vi "QCA - Initialize DUT For AR9880.vi"(8 "error in (no error)":errorcluster, 11 "index":i32) -> (0 "error out":errorcluster, 1 "CmdCount":i32, 2 "Cmd":string, 3 "Command List":string[](array[string]))   [LabVIEW 2012]
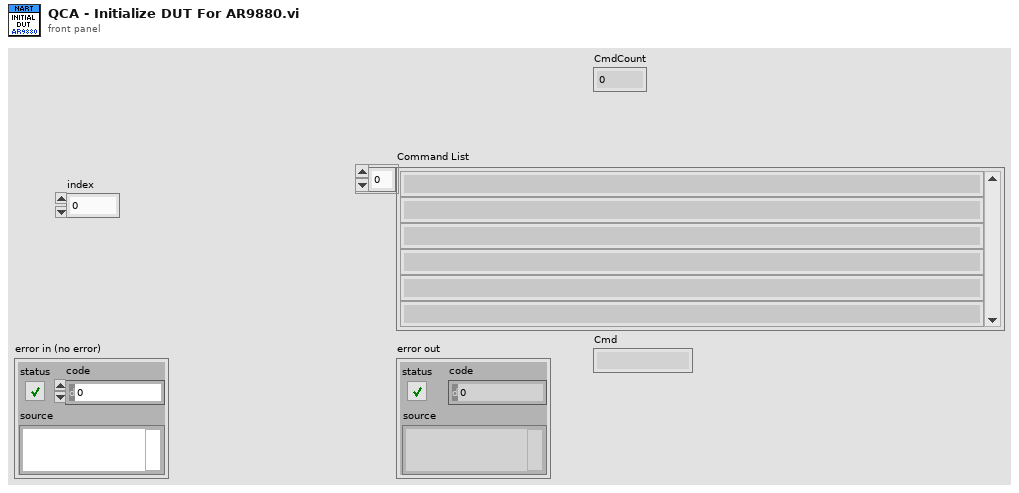
[diagram p1: front panel]
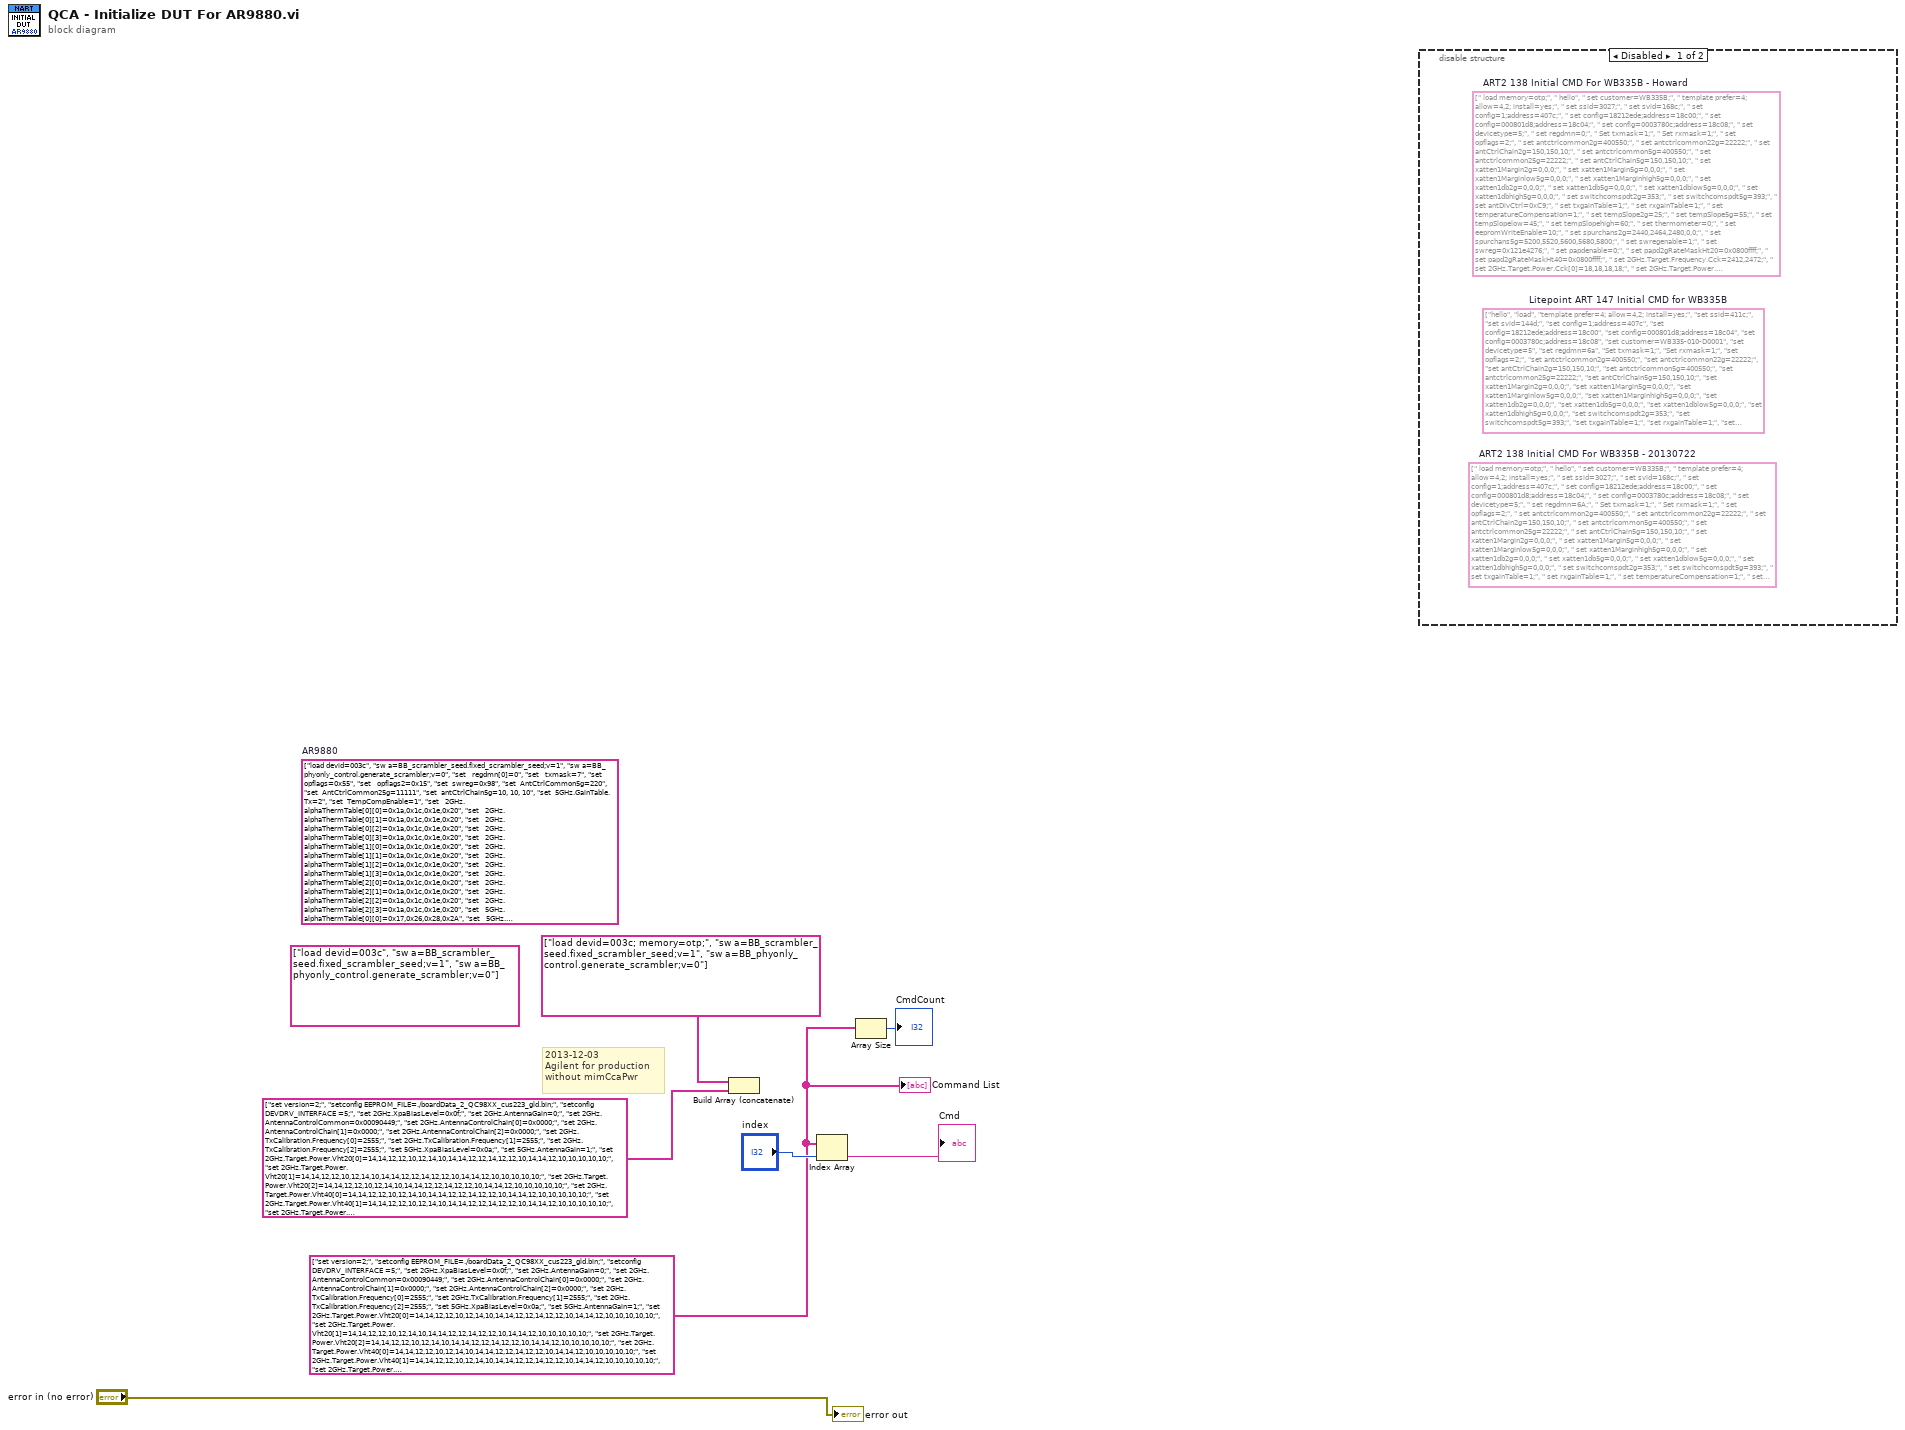
[diagram p0: block diagram]
diagram:
  w1 = string[] ["set version=2;", "setconfig EEPROM_FILE=./boardData_2_QC98XX_cus223_gld.bin;", "setconfig DEVDRV_INTERFACE =5;", "set 2GHz.XpaBiasLevel=0x0f;", "set 2GHz.AntennaGain=0;", "set 2GHz.AntennaControlCommon=0x00090449;", "set 2GHz.AntennaControlChain[0]=0x0000;", "set 2GHz.AntennaControlChain[1]=0x0000;", "set 2GHz.AntennaControlChain[2]=0x0000;", "set 2GHz.TxCalibration.Frequency[0]=2555;", "set 2GHz.TxCalibration.Frequency[1]=2555;", "set 2GHz.TxCalibration.Frequency[2]=2555;", "set 5GHz.XpaBiasLevel=0x0a;", "set 5GHz.AntennaGain=1;", "set 2GHz.Target.Power.Vht20[0]=14,14,12,12,10,12,14,10,14,14,12,12,14,12,12,10,14,14,12,10,10,10,10,10;", "set 2GHz.Target.Power.Vht20[1]=14,14,12,12,10,12,14,10,14,14,12,12,14,12,12,10,14,14,12,10,10,10,10,10;", "set 2GHz.Target.Power.Vht20[2]=14,14,12,12,10,12,14,10,14,14,12,12,14,12,12,10,14,14,12,10,10,10,10,10;", "set 2GHz.Target.Power.Vht40[0]=14,14,12,12,10,12,14,10,14,14,12,12,14,12,12,10,14,14,12,10,10,10,10,10;", "set 2GHz.Target.Power.Vht40[1]=14,14,12,12,10,12,14,10,14,14,12,12,14,12,12,10,14,14,12,10,10,10,10,10;", "set 2GHz.Target.Power.Vht40[2]=14,14,12,12,10,12,14,10,14,14,12,12,14,12,12,10,14,14,12,10,10,10,10,10;", "set regdmn[0]=0;", "set txmask=7;", "set rxmask=7;", "set opflags=0x55;", "set opflags2=0x15;", "set swreg=0x98;", "set AntCtrlCommon5g=220;", "set AntCtrlCommon25g=11111;", "set antCtrlChain5g=10,10,10;", "set 5GHz.GainTable.Tx=2;", "set 5GHz.GainTable.Rx=0;", "set TempCompEnable=1;", "set 2GHz.alphaThermTable[0][0]=0x1a,0x1c,0x1e,0x20;", "set 2GHz.alphaThermTable[0][1]=0x1a,0x1c,0x1e,0x20;", "set 2GHz.alphaThermTable[0][2]=0x1a,0x1c,0x1e,0x20;", "set 2GHz.alphaThermTable[0][3]=0x1a,0x1c,0x1e,0x20;", "set 2GHz.alphaThermTable[1][0]=0x1a,0x1c,0x1e,0x20;", "set 2GHz.alphaThermTable[1][1]=0x1a,0x1c,0x1e,0x20;", "set 2GHz.alphaThermTable[1][2]=0x1a,0x1c,0x1e,0x20;", "set 2GHz.alphaThermTable[1][3]=0x1a,0x1c,0x1e,0x20;", "set 2GHz.alphaThermTable[2][0]=0x1a,0x1c,0x1e,0x20;", "set 2GHz.alphaThermTable[2][1]=0x1a,0x1c,0x1e,0x20;", "set 2GHz.alphaThermTable[2][2]=0x1a,0x1c,0x1e,0x20;", "set 2GHz.alphaThermTable[2][3]=0x1a,0x1c,0x1e,0x20;", "set 5GHz.alphaThermTable[0][0]=0x24,0x24,0x26,0x2C;", "set 5GHz.alphaThermTable[0][1]=0x24,0x24,0x26,0x2C;", "set 5GHz.alphaThermTable[0][2]=0x24,0x24,0x26,0x2C;", "set 5GHz.alphaThermTable[0][3]=0x24,0x24,0x26,0x2C;", "set 5GHz.alphaThermTable[0][4]=0x27,0x26,0x3D,0x3A;", "set 5GHz.alphaThermTable[0][5]=0x27,0x26,0x3D,0x3A;", "set 5GHz.alphaThermTable[0][6]=0x27,0x26,0x3D,0x3A;", "set 5GHz.alphaThermTable[0][7]=0x27,0x26,0x3D,0x3A;", "set 5GHz.alphaThermTable[1][0]=0x24,0x24,0x30,0x34;", "set 5GHz.alphaThermTable[1][1]=0x24,0x24,0x30,0x34;", "set 5GHz.alphaThermTable[1][2]=0x24,0x24,0x30,0x34;", "set 5GHz.alphaThermTable[1][3]=0x24,0x24,0x30,0x34;", "set 5GHz.alphaThermTable[1][4]=0x24,0x24,0x42,0x3E;", "set 5GHz.alphaThermTable[1][5]=0x24,0x24,0x42,0x3E;", "set 5GHz.alphaThermTable[1][6]=0x24,0x24,0x42,0x3E;", "set 5GHz.alphaThermTable[1][7]=0x24,0x24,0x42,0x3E;", "set 5GHz.alphaThermTable[2][0]=0x2B,0x2D,0x21,0x2E;", "set 5GHz.alphaThermTable[2][1]=0x2B,0x2D,0x21,0x2E;", "set 5GHz.alphaThermTable[2][2]=0x2B,0x2D,0x21,0x2E;", "set 5GHz.alphaThermTable[2][3]=0x2B,0x2D,0x21,0x2E;", "set 5GHz.alphaThermTable[2][4]=0x2C,0x2B,0x35,0x39;", "set 5GHz.alphaThermTable[2][5]=0x2C,0x2B,0x35,0x39;", "set 5GHz.alphaThermTable[2][6]=0x2C,0x2B,0x35,0x39;", "set 5GHz.alphaThermTable[2][7]=0x2C,0x2B,0x35,0x39;", "set FeatureEnable.TuningCaps=1;", "set TuningCaps=0x4f,0x4f;", "set antctrlchain5g=0x10;", "set 5GHz.Xatten1Db.Low =0x10,0x15,0x15;", "set 5GHz.Xatten1Db.Mid =0x12,0x15,0x12;", "set 5GHz.Xatten1Db.High =0x12,0x15,0x12;", "set 5GHz.Xatten1Margin.Low =0xa,0xa,0xa;", "set 5GHz.Xatten1Margin.Mid =0xa,0xa,0xa;", "set 5GHz.Xatten1Margin.High =0xa,0xa,0xa;", "set 5GHz.ctl.Index[0]=0x10;", "set 5GHz.ctl.Frequency[0]=5180,5260,5280,5500,5600,5700,5745,5825;", "set 5GHz.ctl.Power[0]=30.5  ,30.5  ,30.5  ,30.5  ,30.5  ,30.5  ,30.5  ,30;", "set 5GHz.ctl.BandEdge[0]=0   ,0   ,0   ,0   ,0   ,0   ,0   ,0;", "set 5GHz.ctl.Index[1]=0x16;", "set 5GHz.ctl.Frequency[1]=5180,5260,5280,5500,5520,5700,5745,5825;", "set 5GHz.ctl.Power[1]=30.5  ,30.5  ,30.5  ,30.5  ,30.5  ,30.5  ,30.5  ,30;", "set 5GHz.ctl.BandEdge[1]=0   ,0   ,0   ,0   ,0   ,0   ,0   ,0;", "set 5GHz.ctl.Index[2]=0x18;", "set 5GHz.ctl.Frequency[2]=5190,5230,5270,5310,5510,5550,5670,5755;", "set 5GHz.ctl.Power[2]=30  ,30.5  ,30  ,30.5  ,30.5  ,30.5  ,30.5  ,30.5;", "set 5GHz.ctl.BandEdge[2]=0   ,0   ,0   ,0   ,0   ,0   ,0   ,0;", "set 5GHz.ctl.Index[3]=0x19;", "set 5GHz.ctl.Frequency[3]=5180,5260,5280,5500,5520,5700,0,0;", "set 5GHz.ctl.Power[3]=30.5  ,30.5  ,30.5  ,30.5  ,30.5  ,30.5  ,0,0;", "set 5GHz.ctl.BandEdge[3]=0   ,0   ,0   ,0   ,0   ,0   ,0,0;", "set 5GHz.ctl.Index[6]=0x40;", "set 5GHz.ctl.Frequency[6]=5180,5200,5260,5320,5500,5700,6075,6075;", "set 5GHz.ctl.Power[6]=30  ,30.5  ,30.5  ,30  ,30.5  ,30  ,30  ,30;", "set 5GHz.ctl.BandEdge[6]=0   ,0   ,0   ,0   ,0   ,0   ,0   ,0;", "set 5GHz.ctl.Index[7]=0x46;", "set 5GHz.ctl.Frequency[7]=5180,5260,5500,5700,6075,6075,6075,6075;", "set 5GHz.ctl.Power[7]=30.5  ,30.5  ,30.5  ,30  ,30  ,30  ,30  ,30;", "set 5GHz.ctl.BandEdge[7]=0   ,0   ,0   ,0   ,0   ,0   ,0   ,0;", "set 5GHz.ctl.Index[8]=0x48;", "set 5GHz.ctl.Frequency[8]=5190,5270,5310,5510,5590,5670,6075,6075;", "set 5GHz.ctl.Power[8]=30.5  ,30.5  ,30.5  ,30.5  ,30.5  ,30  ,30  ,30;", "set 5GHz.ctl.BandEdge[8]=0   ,0   ,0   ,0   ,0   ,0   ,0   ,0;", "set 5GHz.ctl.Index[9]=0x49;", "set 5GHz.ctl.Frequency[9]=5180,5260,5500,5700,0,0,0,0;", "set 5GHz.ctl.Power[9]=30.5  ,30.5  ,30.5  ,30  ,0,0,0,0;", "set 5GHz.ctl.BandEdge[9]=0   ,0   ,0   ,0   ,0,0,0,0;", "set 5GHz.ctl.Index[12]=0x30;", "set 5GHz.ctl.Frequency[12]=5180,5200,5220,5260,5500,5600,5700,5745;", "set 5GHz.ctl.Power[12]=30.5  ,30.5  ,30.5  ,30.5  ,30.5  ,30.5  ,30.5  ,30.5;", "set 5GHz.ctl.BandEdge[12]=0   ,0   ,0   ,0   ,0   ,0   ,0   ,0;", "set 5GHz.ctl.Index[13]=0x36;", "set 5GHz.ctl.Frequency[13]=5180,5260,5320,5500,5560,5700,5745,5825;", "set 5GHz.ctl.Power[13]=30.5  ,30.5  ,30  ,30.5  ,30.5  ,30.5  ,30.5  ,30;", "set 5GHz.ctl.BandEdge[13]=0   ,0   ,0   ,0   ,0   ,0   ,0   ,0;", "set 5GHz.ctl.Index[14]=0x38;", "set 5GHz.ctl.Frequency[14]=5190,5230,5270,5510,5550,5670,5755,5795;", "set 5GHz.ctl.Power[14]=30.5  ,30  ,30.5  ,30.5  ,30.5  ,30.5  ,30  ,30.5;", "set 5GHz.ctl.BandEdge[14]=0   ,0   ,0   ,0   ,0   ,0   ,0   ,0;", "set 5GHz.ctl.Index[15]=0x39;", "set 5GHz.ctl.Frequency[15]=5180,5260,5320,5500,5560,5700,0,0;", "set 5GHz.ctl.Power[15]=30.5  ,30.5  ,30  ,30.5  ,30.5  ,30.5  ,0,0;", "set 5GHz.ctl.BandEdge[15]=0   ,0   ,0   ,0   ,0   ,0   ,0,0;", "set 5GHz.Target.Power.Legacy[0]=13.5,13.5,13.5,13.5;", "set 5GHz.Target.Power.Legacy[1]=13.5,13.5,13.5,13.5;", "set 5GHz.Target.Power.Legacy[2]=13.5,13.5,13.5,13.5;", "set 5GHz.Target.Power.Legacy[3]=19,18,17,17;", "set 5GHz.Target.Power.Legacy[4]=19,18,17,17;", "set 5GHz.Target.Power.Legacy[5]=19,18,17,17;", "set 5GHz.Target.Frequency.Vht20=5180,5240,5320,5500,5600,5745;", "set 5GHz.Target.Power.Vht20[0]=13.5,13.5,13.5,13.5,13.5,13.5,13.5,13.5,13.5,13.5,13.5,13.5,13.5,13.5,13.5,13.5,13.5,13.5,13.5,13.5,13.5,13.5,13.5,13.5;", "set 5GHz.Target.Power.Vht20[1]=13.5,13.5,13.5,13.5,13.5,13.5,13.5,13.5,13.5,13.5,13.5,13.5,13.5,13.5,13.5,13.5,13.5,13.5,13.5,13.5,13.5,13.5,13.5,13.5;", "set 5GHz.Target.Power.Vht20[2]=13.5,13.5,13.5,13.5,13.5,13.5,13.5,13.5,13.5,13.5,13.5,13.5,13.5,13.5,13.5,13.5,13.5,13.5,13.5,13.5,13.5,13.5,13.5,13.5;", "set 5GHz.Target.Power.Vht20[3]=19,19,18,17,17,16,14,14,19,19,18,17,17,16,14,14,19,19,18,17,17,16,14,14;", "set 5GHz.Target.Power.Vht20[4]=19,19,18,17,17,16,14,14,19,19,18,17,17,16,14,14,19,19,18,17,17,16,14,14;", "set 5GHz.Target.Power.Vht20[5]=19,19,18,17,17,16,14,14,19,19,18,17,17,16,14,14,19,19,18,17,17,16,14,14;", "set 5GHz.Target.Frequency.Vht40=5180,5240,5320,5500,5600,5745;", "set 5GHz.Target.Power.Vht40[0]=13.5,13.5,13.5,13.5,13.5,13.5,13.5,13.5,13.5,13.5,13.5,13.5,13.5,13.5,13.5,13.5,13.5,13.5,13.5,13.5,13.5,13.5,13.5,13.5;", "set 5GHz.Target.Power.Vht40[1]=13.5,13.5,13.5,13.5,13.5,13.5,13.5,13.5,13.5,13.5,13.5,13.5,13.5,13.5,13.5,13.5,13.5,13.5,13.5,13.5,13.5,13.5,13.5,13.5;", "set 5GHz.Target.Power.Vht40[2]=13.5,13.5,13.5,13.5,13.5,13.5,13.5,13.5,13.5,13.5,13.5,13.5,13.5,13.5,13.5,13.5,13.5,13.5,13.5,13.5,13.5,13.5,13.5,13.5;", "set 5GHz.Target.Power.Vht40[3]=19,19,18,17,17,16,14,14,19,19,18,17,17,16,14,14,19,19,18,17,17,16,14,14;", "set 5GHz.Target.Power.Vht40[4]=19,19,18,17,17,16,14,14,19,19,18,17,17,16,14,14,19,19,18,17,17,16,14,14;", "set 5GHz.Target.Power.Vht40[5]=19,19,18,17,17,16,14,14,19,19,18,17,17,16,14,14,19,19,18,17,17,16,14,14;", "set 5GHz.Target.Frequency.Vht80=5180,5240,5320,5500,5600,5745;", "set 5GHz.Target.Power.Vht80[0]=13.5,13.5,13.5,13.5,13.5,13.5,13.5,13.5,13.5,13.5,13.5,13.5,13.5,13.5,13.5,13.5,13.5,13.5,13.5,13.5,13.5,13.5,13.5,13.5;", "set 5GHz.Target.Power.Vht80[1]=13.5,13.5,13.5,13.5,13.5,13.5,13.5,13.5,13.5,13.5,13.5,13.5,13.5,13.5,13.5,13.5,13.5,13.5,13.5,13.5,13.5,13.5,13.5,13.5;", "set 5GHz.Target.Power.Vht80[2]=13.5,13.5,13.5,13.5,13.5,13.5,13.5,13.5,13.5,13.5,13.5,13.5,13.5,13.5,13.5,13.5,13.5,13.5,13.5,13.5,13.5,13.5,13.5,13.5;", "set 5GHz.Target.Power.Vht80[3]=19,19,18,17,17,16,14,14,19,19,18,17,17,16,14,14,19,19,18,17,17,16,14,14;", "set 5GHz.Target.Power.Vht80[4]=19,19,18,17,17,16,14,14,19,19,18,17,17,16,14,14,19,19,18,17,17,16,14,14;", "set 5GHz.Target.Power.Vht80[5]=19,19,18,17,17,16,14,14,19,19,18,17,17,16,14,14,19,19,18,17,17,16,14,14;", "setcal dll=cal-2p;", "setcal scheme=2;", "setcal PowerGoalMode=1;", "setcal 5gfreq=5180,5240,5320,5520,5640,5745,5785,5825;", "setcal 5gGainIndex1Ch0=9,9,9,9,9,9,10,10;", "setcal 5gGainIndex1Ch1=9,9,9,9,9,9,10,10;", "setcal 5gGainIndex1Ch2=9,9,9,9,9,9,10,10;", "setcal 5gDacGain1=0,0,0,0,0,0,0,0;", "setcal 5gPowerGoal1=14.0,14.0,14.0,14.0,14.0,14.0,14.0,14.0;", "setcal 5gGainIndex2Ch0=12,12,12,12,12,12,13,13;", "setcal 5gGainIndex2Ch1=12,12,12,12,12,12,13,13;", "setcal 5gGainIndex2Ch2=12,12,12,12,12,12,13,13;", "setcal 5gDacGain2=-6,-6,-6,-6,-6,-6,-6,-6;", "setcal 5gPowerGoal2=14.0,14.0,14.0,14.0,14.0,14.0,14.0,14.0;", "set customer=cus223-022-n0624;", "set 5GHz.Target.Frequency.Legacy[0]=5180;", "set 5GHz.Target.Frequency.Legacy[1]=5240;", "set 5GHz.Target.Frequency.Legacy[2]=5320;", "set 5GHz.Target.Frequency.Legacy[3]=5500;", "set 5GHz.Target.Frequency.Legacy[4]=5600;", "set 5GHz.Target.Frequency.Legacy[5]=5745;"] ("最终指令")
  (unwired) string[] ["load devid=003c", "sw a=BB_scrambler_seed.fixed_scrambler_seed;v=1", "sw a=BB_phyonly_control.generate_scrambler;v=0"]
  (unwired) string[] ["load devid=003c", "sw a=BB_scrambler_seed.fixed_scrambler_seed;v=1", "sw a=BB_phyonly_control.generate_scrambler;v=0", "set   regdmn[0]=0", "set   txmask=7", "set   opflags=0x55", "set   opflags2=0x15", "set  swreg=0x98", "set  AntCtrlCommon5g=220", "set  AntCtrlCommon25g=11111", "set  antCtrlChain5g=10, 10, 10", "set  5GHz.GainTable.Tx=2", "set  TempCompEnable=1", "set   2GHz.alphaThermTable[0][0]=0x1a,0x1c,0x1e,0x20", "set   2GHz.alphaThermTable[0][1]=0x1a,0x1c,0x1e,0x20", "set   2GHz.alphaThermTable[0][2]=0x1a,0x1c,0x1e,0x20", "set   2GHz.alphaThermTable[0][3]=0x1a,0x1c,0x1e,0x20", "set   2GHz.alphaThermTable[1][0]=0x1a,0x1c,0x1e,0x20", "set   2GHz.alphaThermTable[1][1]=0x1a,0x1c,0x1e,0x20", "set   2GHz.alphaThermTable[1][2]=0x1a,0x1c,0x1e,0x20", "set   2GHz.alphaThermTable[1][3]=0x1a,0x1c,0x1e,0x20", "set   2GHz.alphaThermTable[2][0]=0x1a,0x1c,0x1e,0x20", "set   2GHz.alphaThermTable[2][1]=0x1a,0x1c,0x1e,0x20", "set   2GHz.alphaThermTable[2][2]=0x1a,0x1c,0x1e,0x20", "set   2GHz.alphaThermTable[2][3]=0x1a,0x1c,0x1e,0x20", "set   5GHz.alphaThermTable[0][0]=0x17,0x26,0x28,0x2A", "set   5GHz.alphaThermTable[0][1]=0x1C,0x26,0x2A,0x2C", "set   5GHz.alphaThermTable[0][2]=0x28,0x2D,0x31,0x33", "set   5GHz.alphaThermTable[0][3]=0x25,0x30,0x35,0x35", "set   5GHz.alphaThermTable[0][4]=0x28,0x30,0x31,0x35", "set   5GHz.alphaThermTable[0][5]=0x2E,0x30,0x37,0x37", "set   5GHz.alphaThermTable[0][6]=0x24,0x33,0x36,0x37\nset   5GHz.alphaThermTable[0][6]=0x24,0x33,0x36,0x37", "set   5GHz.alphaThermTable[0][7]=0x2C,0x34,0x38,0x38", "set   5GHz.alphaThermTable[1][0]=0x17,0x26,0x28,0x2A", "set   5GHz.alphaThermTable[1][1]=0x1C,0x26,0x2A,0x2C", "set   5GHz.alphaThermTable[1][2]=0x28,0x2D,0x31,0x33", "set   5GHz.alphaThermTable[1][3]=0x25,0x30,0x35,0x35", "set   5GHz.alphaThermTable[1][4]=0x28,0x30,0x31,0x35", "set   5GHz.alphaThermTable[1][5]=0x2E,0x30,0x37,0x37", "set   5GHz.alphaThermTable[1][6]=0x24,0x33,0x36,0x37", "set   5GHz.alphaThermTable[1][7]=0x2C,0x34,0x38,0x38", "set   5GHz.alphaThermTable[2][0]=0x17,0x26,0x28,0x2A", "set   5GHz.alphaThermTable[2][1]=0x1C,0x26,0x2A,0x2C", "set   5GHz.alphaThermTable[2][2]=0x28,0x2D,0x31,0x33", "set   5GHz.alphaThermTable[2][3]=0x25,0x30,0x35,0x35", "set   5GHz.alphaThermTable[2][4]=0x28,0x30,0x31,0x35", "set   5GHz.alphaThermTable[2][5]=0x2E,0x30,0x37,0x37", "set   5GHz.alphaThermTable[2][6]=0x24,0x33,0x36,0x37", "set   5GHz.alphaThermTable[2][7]=0x2C,0x34,0x38,0x38", "set FeatureEnable.TuningCaps=1", "set TuningCaps=0x4f,0x4f", "set  antctrlchain5g=0x10", "set  5GHz.Xatten1Db.Low = 0x18", "set  5GHz.Xatten1Db.Mid = 0x18", "set  5GHz.Xatten1Db.High = 0x18", "set  5GHz.Xatten1Margin.Low = 0x8", "set  5GHz.Xatten1Margin.Mid = 0x8", "set  5GHz.Xatten1Margin.High = 0x8", "set   5GHz.Target.Frequency.Legacy=5180,5240,5320,5500,5600,5745", "set  5GHz.Target.Power.Legacy[0]=17,17,17,15", "set  5GHz.Target.Power.Legacy[1]=17,17,17,15", "set  5GHz.Target.Power.Legacy[2]=20,20,20,18", "set  5GHz.Target.Power.Legacy[3]=20,20,20,18", "set  5GHz.Target.Power.Legacy[4]=20,20,20,18", "set  5GHz.Target.Power.Legacy[5]=20,20,20,18", "set   5GHz.Target.Frequency.Vht20=5180,5240,5320,5500,5600,5745", "set  5GHz.Target.Power.Vht20[0]=17,17,17,17,17,15,14,13,17,17,17,17,17,15,14,13,17,17,17,17,17,15,14,13", "set  5GHz.Target.Power.Vht20[1]=17,17,17,17,17,15,14,13,17,17,17,17,17,15,14,13,17,17,17,17,17,15,14,13", "set  5GHz.Target.Power.Vht20[2]=20,20,20,20,20,18,16,13,20,20,20,20,20,18,16,13,20,20,20,20,20,18,16,13", "set  5GHz.Target.Power.Vht20[3]=20,20,20,20,20,18,16,13,20,20,20,20,20,18,16,13,20,20,20,20,20,18,16,13", "set  5GHz.Target.Power.Vht20[4]=20,20,20,20,20,18,16,13,20,20,20,20,20,18,16,13,20,20,20,20,20,18,16,13", "set  5GHz.Target.Power.Vht20[5]=20,20,20,20,20,18,16,13,20,20,20,20,20,18,16,13,20,20,20,20,20,18,16,13", "set  5GHz.Target.Frequency.Vht40=5180,5240,5320,5500,5600,5745", "set  5GHz.Target.Power.Vht40[0]=17,17,17,17,17,15,14,13,17,17,17,17,17,15,14,13,17,17,17,17,17,15,14,13", "set  5GHz.Target.Power.Vht40[1]=17,17,17,17,17,15,14,13,17,17,17,17,17,15,14,13,17,17,17,17,17,15,14,13", "set  5GHz.Target.Power.Vht40[2]=20,20,20,20,20,18,16,13,20,20,20,20,20,18,16,13,20,20,20,20,20,18,16,13", "set  5GHz.Target.Power.Vht40[3]=20,20,20,20,20,18,16,13,20,20,20,20,20,18,16,13,20,20,20,20,20,18,16,13", "set  5GHz.Target.Power.Vht40[4]=20,20,20,20,20,18,16,13,20,20,20,20,20,18,16,13,20,20,20,20,20,18,16,13", "set  5GHz.Target.Power.Vht40[5]=20,20,20,20,20,18,16,13,20,20,20,20,20,18,16,13,20,20,20,20,20,18,16,13", "set  5GHz.Target.Frequency.Vht80=5180,5240,5320,5500,5600,5745", "set  5GHz.Target.Power.Vht80[0]=17,17,17,17,17,15,14,13,17,17,17,17,17,15,14,13,17,17,17,17,17,15,14,13", "set  5GHz.Target.Power.Vht80[1]=17,17,17,17,17,15,14,13,17,17,17,17,17,15,14,13,17,17,17,17,17,15,14,13", "set  5GHz.Target.Power.Vht80[2]=20,20,20,20,20,18,16,13,20,20,20,20,20,18,16,13,20,20,20,20,20,18,16,13", "set  5GHz.Target.Power.Vht80[3]=20,20,20,20,20,18,16,13,20,20,20,20,20,18,16,13,20,20,20,20,20,18,16,13", "set  5GHz.Target.Power.Vht80[4]=20,20,20,20,20,18,16,13,20,20,20,20,20,18,16,13,20,20,20,20,20,18,16,13", "set  5GHz.Target.Power.Vht80[5]=20,20,20,20,20,18,16,13,20,20,20,20,20,18,16,13,20,20,20,20,20,18,16,13", "setcal  dll=cal-2p", "setcal  scheme=2", "setcal  PowerGoalMode=1", "setcal  5gfreq=5180,5240,5320,5520,5640,5745,5785,5825", "setcal  5gGainIndex1Ch0=9,9,9,9,9,9,10,10", "setcal  5gGainIndex1Ch1=9,9,9,9,9,9,10,10", "setcal  5gGainIndex1Ch2=9,9,9,9,9,9,10,10", "setcal  5gDacGain1=0,0,0,0,0,0,0,0", "setcal  5gPowerGoal1=14.0,14.0,14.0,14.0,14.0,14.0,14.0,14.0", "setcal  5gGainIndex2Ch0=12,12,12,12,12,12,13,13", "setcal  5gGainIndex2Ch1=12,12,12,12,12,12,13,13", "setcal  5gGainIndex2Ch2=12,12,12,12,12,12,13,13", "setcal  5gDacGain2=-6,-6,-6,-6,-6,-6,-6,-6", "setcal  5gPowerGoal2=14.0,14.0,14.0,14.0,14.0,14.0,14.0,14.0", "set ssid=3223;", "set svid=168C;"]  # AR9880
  # "2013-12-03 \nAgilent for production\nwithout mimCcaPwr"
  n1 = Build Array (concatenate)(string[] ["load devid=003c; memory=otp;", "sw a=BB_scrambler_seed.fixed_scrambler_seed;v=1", "sw a=BB_phyonly_control.generate_scrambler;v=0"], string[] ["set version=2;", "setconfig EEPROM_FILE=./boardData_2_QC98XX_cus223_gld.bin;", "setconfig DEVDRV_INTERFACE =5;", "set 2GHz.XpaBiasLevel=0x0f;", "set 2GHz.AntennaGain=0;", "set 2GHz.AntennaControlCommon=0x00090449;", "set 2GHz.AntennaControlChain[0]=0x0000;", "set 2GHz.AntennaControlChain[1]=0x0000;", "set 2GHz.AntennaControlChain[2]=0x0000;", "set 2GHz.TxCalibration.Frequency[0]=2555;", "set 2GHz.TxCalibration.Frequency[1]=2555;", "set 2GHz.TxCalibration.Frequency[2]=2555;", "set 5GHz.XpaBiasLevel=0x0a;", "set 5GHz.AntennaGain=1;", "set 2GHz.Target.Power.Vht20[0]=14,14,12,12,10,12,14,10,14,14,12,12,14,12,12,10,14,14,12,10,10,10,10,10;", "set 2GHz.Target.Power.Vht20[1]=14,14,12,12,10,12,14,10,14,14,12,12,14,12,12,10,14,14,12,10,10,10,10,10;", "set 2GHz.Target.Power.Vht20[2]=14,14,12,12,10,12,14,10,14,14,12,12,14,12,12,10,14,14,12,10,10,10,10,10;", "set 2GHz.Target.Power.Vht40[0]=14,14,12,12,10,12,14,10,14,14,12,12,14,12,12,10,14,14,12,10,10,10,10,10;", "set 2GHz.Target.Power.Vht40[1]=14,14,12,12,10,12,14,10,14,14,12,12,14,12,12,10,14,14,12,10,10,10,10,10;", "set 2GHz.Target.Power.Vht40[2]=14,14,12,12,10,12,14,10,14,14,12,12,14,12,12,10,14,14,12,10,10,10,10,10;", "set regdmn[0]=0;", "set txmask=7;", "set rxmask=7;", "set opflags=0x55;", "set opflags2=0x15;", "set swreg=0x98;", "set AntCtrlCommon5g=220;", "set AntCtrlCommon25g=11111;", "set antCtrlChain5g=10,10,10;", "set 5GHz.GainTable.Tx=2;", "set 5GHz.GainTable.Rx=0;", "set TempCompEnable=1;", "set 2GHz.alphaThermTable[0][0]=0x1a,0x1c,0x1e,0x20;", "set 2GHz.alphaThermTable[0][1]=0x1a,0x1c,0x1e,0x20;", "set 2GHz.alphaThermTable[0][2]=0x1a,0x1c,0x1e,0x20;", "set 2GHz.alphaThermTable[0][3]=0x1a,0x1c,0x1e,0x20;", "set 2GHz.alphaThermTable[1][0]=0x1a,0x1c,0x1e,0x20;", "set 2GHz.alphaThermTable[1][1]=0x1a,0x1c,0x1e,0x20;", "set 2GHz.alphaThermTable[1][2]=0x1a,0x1c,0x1e,0x20;", "set 2GHz.alphaThermTable[1][3]=0x1a,0x1c,0x1e,0x20;", "set 2GHz.alphaThermTable[2][0]=0x1a,0x1c,0x1e,0x20;", "set 2GHz.alphaThermTable[2][1]=0x1a,0x1c,0x1e,0x20;", "set 2GHz.alphaThermTable[2][2]=0x1a,0x1c,0x1e,0x20;", "set 2GHz.alphaThermTable[2][3]=0x1a,0x1c,0x1e,0x20;", "set 5GHz.alphaThermTable[0][0]=0x24,0x24,0x26,0x2C;", "set 5GHz.alphaThermTable[0][1]=0x24,0x24,0x26,0x2C;", "set 5GHz.alphaThermTable[0][2]=0x24,0x24,0x26,0x2C;", "set 5GHz.alphaThermTable[0][3]=0x24,0x24,0x26,0x2C;", "set 5GHz.alphaThermTable[0][4]=0x27,0x26,0x3D,0x3A;", "set 5GHz.alphaThermTable[0][5]=0x27,0x26,0x3D,0x3A;", "set 5GHz.alphaThermTable[0][6]=0x27,0x26,0x3D,0x3A;", "set 5GHz.alphaThermTable[0][7]=0x27,0x26,0x3D,0x3A;", "set 5GHz.alphaThermTable[1][0]=0x24,0x24,0x30,0x34;", "set 5GHz.alphaThermTable[1][1]=0x24,0x24,0x30,0x34;", "set 5GHz.alphaThermTable[1][2]=0x24,0x24,0x30,0x34;", "set 5GHz.alphaThermTable[1][3]=0x24,0x24,0x30,0x34;", "set 5GHz.alphaThermTable[1][4]=0x24,0x24,0x42,0x3E;", "set 5GHz.alphaThermTable[1][5]=0x24,0x24,0x42,0x3E;", "set 5GHz.alphaThermTable[1][6]=0x24,0x24,0x42,0x3E;", "set 5GHz.alphaThermTable[1][7]=0x24,0x24,0x42,0x3E;", "set 5GHz.alphaThermTable[2][0]=0x2B,0x2D,0x21,0x2E;", "set 5GHz.alphaThermTable[2][1]=0x2B,0x2D,0x21,0x2E;", "set 5GHz.alphaThermTable[2][2]=0x2B,0x2D,0x21,0x2E;", "set 5GHz.alphaThermTable[2][3]=0x2B,0x2D,0x21,0x2E;", "set 5GHz.alphaThermTable[2][4]=0x2C,0x2B,0x35,0x39;", "set 5GHz.alphaThermTable[2][5]=0x2C,0x2B,0x35,0x39;", "set 5GHz.alphaThermTable[2][6]=0x2C,0x2B,0x35,0x39;", "set 5GHz.alphaThermTable[2][7]=0x2C,0x2B,0x35,0x39;", "set FeatureEnable.TuningCaps=1;", "set TuningCaps=0x50,0x50;", "set antctrlchain5g=0x10;", "set 5GHz.Xatten1Db.Low =0x10,0x15,0x15;", "set 5GHz.Xatten1Db.Mid =0x12,0x15,0x12;", "set 5GHz.Xatten1Db.High =0x12,0x15,0x12;", "set 5GHz.Xatten1Margin.Low =0xa,0xa,0xa;", "set 5GHz.Xatten1Margin.Mid =0xa,0xa,0xa;", "set 5GHz.Xatten1Margin.High =0xa,0xa,0xa;", "set 5GHz.ctl.Index[0]=0x10;", "set 5GHz.ctl.Frequency[0]=5180,5260,5280,5500,5600,5700,5745,5825;", "set 5GHz.ctl.Power[0]=30.5  ,30.5  ,30.5  ,30.5  ,30.5  ,30.5  ,30.5  ,30;", "set 5GHz.ctl.BandEdge[0]=0   ,0   ,0   ,0   ,0   ,0   ,0   ,0;", "set 5GHz.ctl.Index[1]=0x16;", "set 5GHz.ctl.Frequency[1]=5180,5260,5280,5500,5520,5700,5745,5825;", "set 5GHz.ctl.Power[1]=30.5  ,30.5  ,30.5  ,30.5  ,30.5  ,30.5  ,30.5  ,30;", "set 5GHz.ctl.BandEdge[1]=0   ,0   ,0   ,0   ,0   ,0   ,0   ,0;", "set 5GHz.ctl.Index[2]=0x18;", "set 5GHz.ctl.Frequency[2]=5190,5230,5270,5310,5510,5550,5670,5755;", "set 5GHz.ctl.Power[2]=30  ,30.5  ,30  ,30.5  ,30.5  ,30.5  ,30.5  ,30.5;", "set 5GHz.ctl.BandEdge[2]=0   ,0   ,0   ,0   ,0   ,0   ,0   ,0;", "set 5GHz.ctl.Index[3]=0x19;", "set 5GHz.ctl.Frequency[3]=5180,5260,5280,5500,5520,5700,0,0;", "set 5GHz.ctl.Power[3]=30.5  ,30.5  ,30.5  ,30.5  ,30.5  ,30.5  ,0,0;", "set 5GHz.ctl.BandEdge[3]=0   ,0   ,0   ,0   ,0   ,0   ,0,0;", "set 5GHz.ctl.Index[6]=0x40;", "set 5GHz.ctl.Frequency[6]=5180,5200,5260,5320,5500,5700,6075,6075;", "set 5GHz.ctl.Power[6]=30  ,30.5  ,30.5  ,30  ,30.5  ,30  ,30  ,30;", "set 5GHz.ctl.BandEdge[6]=0   ,0   ,0   ,0   ,0   ,0   ,0   ,0;", "set 5GHz.ctl.Index[7]=0x46;", "set 5GHz.ctl.Frequency[7]=5180,5260,5500,5700,6075,6075,6075,6075;", "set 5GHz.ctl.Power[7]=30.5  ,30.5  ,30.5  ,30  ,30  ,30  ,30  ,30;", "set 5GHz.ctl.BandEdge[7]=0   ,0   ,0   ,0   ,0   ,0   ,0   ,0;", "set 5GHz.ctl.Index[8]=0x48;", "set 5GHz.ctl.Frequency[8]=5190,5270,5310,5510,5590,5670,6075,6075;", "set 5GHz.ctl.Power[8]=30.5  ,30.5  ,30.5  ,30.5  ,30.5  ,30  ,30  ,30;", "set 5GHz.ctl.BandEdge[8]=0   ,0   ,0   ,0   ,0   ,0   ,0   ,0;", "set 5GHz.ctl.Index[9]=0x49;", "set 5GHz.ctl.Frequency[9]=5180,5260,5500,5700,0,0,0,0;", "set 5GHz.ctl.Power[9]=30.5  ,30.5  ,30.5  ,30  ,0,0,0,0;", "set 5GHz.ctl.BandEdge[9]=0   ,0   ,0   ,0   ,0,0,0,0;", "set 5GHz.ctl.Index[12]=0x30;", "set 5GHz.ctl.Frequency[12]=5180,5200,5220,5260,5500,5600,5700,5745;", "set 5GHz.ctl.Power[12]=30.5  ,30.5  ,30.5  ,30.5  ,30.5  ,30.5  ,30.5  ,30.5;", "set 5GHz.ctl.BandEdge[12]=0   ,0   ,0   ,0   ,0   ,0   ,0   ,0;", "set 5GHz.ctl.Index[13]=0x36;", "set 5GHz.ctl.Frequency[13]=5180,5260,5320,5500,5560,5700,5745,5825;", "set 5GHz.ctl.Power[13]=30.5  ,30.5  ,30  ,30.5  ,30.5  ,30.5  ,30.5  ,30;", "set 5GHz.ctl.BandEdge[13]=0   ,0   ,0   ,0   ,0   ,0   ,0   ,0;", "set 5GHz.ctl.Index[14]=0x38;", "set 5GHz.ctl.Frequency[14]=5190,5230,5270,5510,5550,5670,5755,5795;", "set 5GHz.ctl.Power[14]=30.5  ,30  ,30.5  ,30.5  ,30.5  ,30.5  ,30  ,30.5;", "set 5GHz.ctl.BandEdge[14]=0   ,0   ,0   ,0   ,0   ,0   ,0   ,0;", "set 5GHz.ctl.Index[15]=0x39;", "set 5GHz.ctl.Frequency[15]=5180,5260,5320,5500,5560,5700,0,0;", "set 5GHz.ctl.Power[15]=30.5  ,30.5  ,30  ,30.5  ,30.5  ,30.5  ,0,0;", "set 5GHz.ctl.BandEdge[15]=0   ,0   ,0   ,0   ,0   ,0   ,0,0;", "set 5GHz.Target.Power.Legacy[0]=13.5,13.5,13.5,13.5;", "set 5GHz.Target.Power.Legacy[1]=13.5,13.5,13.5,13.5;", "set 5GHz.Target.Power.Legacy[2]=13.5,13.5,13.5,13.5;", "set 5GHz.Target.Power.Legacy[3]=19,18,17,17;", "set 5GHz.Target.Power.Legacy[4]=19,18,17,17;", "set 5GHz.Target.Power.Legacy[5]=19,18,17,17;", "set 5GHz.Target.Frequency.Vht20=5180,5240,5320,5500,5600,5745;", "set 5GHz.Target.Power.Vht20[0]=13.5,13.5,13.5,13.5,13.5,13.5,13.5,13.5,13.5,13.5,13.5,13.5,13.5,13.5,13.5,13.5,13.5,13.5,13.5,13.5,13.5,13.5,13.5,13.5;", "set 5GHz.Target.Power.Vht20[1]=13.5,13.5,13.5,13.5,13.5,13.5,13.5,13.5,13.5,13.5,13.5,13.5,13.5,13.5,13.5,13.5,13.5,13.5,13.5,13.5,13.5,13.5,13.5,13.5;", "set 5GHz.Target.Power.Vht20[2]=13.5,13.5,13.5,13.5,13.5,13.5,13.5,13.5,13.5,13.5,13.5,13.5,13.5,13.5,13.5,13.5,13.5,13.5,13.5,13.5,13.5,13.5,13.5,13.5;", "set 5GHz.Target.Power.Vht20[3]=19,19,18,17,17,16,14,14,19,19,18,17,17,16,14,14,19,19,18,17,17,16,14,14;", "set 5GHz.Target.Power.Vht20[4]=19,19,18,17,17,16,14,14,19,19,18,17,17,16,14,14,19,19,18,17,17,16,14,14;", "set 5GHz.Target.Power.Vht20[5]=19,19,18,17,17,16,14,14,19,19,18,17,17,16,14,14,19,19,18,17,17,16,14,14;", "set 5GHz.Target.Frequency.Vht40=5180,5240,5320,5500,5600,5745;", "set 5GHz.Target.Power.Vht40[0]=13.5,13.5,13.5,13.5,13.5,13.5,13.5,13.5,13.5,13.5,13.5,13.5,13.5,13.5,13.5,13.5,13.5,13.5,13.5,13.5,13.5,13.5,13.5,13.5;", "set 5GHz.Target.Power.Vht40[1]=13.5,13.5,13.5,13.5,13.5,13.5,13.5,13.5,13.5,13.5,13.5,13.5,13.5,13.5,13.5,13.5,13.5,13.5,13.5,13.5,13.5,13.5,13.5,13.5;", "set 5GHz.Target.Power.Vht40[2]=13.5,13.5,13.5,13.5,13.5,13.5,13.5,13.5,13.5,13.5,13.5,13.5,13.5,13.5,13.5,13.5,13.5,13.5,13.5,13.5,13.5,13.5,13.5,13.5;", "set 5GHz.Target.Power.Vht40[3]=19,19,18,17,17,16,14,14,19,19,18,17,17,16,14,14,19,19,18,17,17,16,14,14;", "set 5GHz.Target.Power.Vht40[4]=19,19,18,17,17,16,14,14,19,19,18,17,17,16,14,14,19,19,18,17,17,16,14,14;", "set 5GHz.Target.Power.Vht40[5]=19,19,18,17,17,16,14,14,19,19,18,17,17,16,14,14,19,19,18,17,17,16,14,14;", "set 5GHz.Target.Frequency.Vht80=5180,5240,5320,5500,5600,5745;", "set 5GHz.Target.Power.Vht80[0]=13.5,13.5,13.5,13.5,13.5,13.5,13.5,13.5,13.5,13.5,13.5,13.5,13.5,13.5,13.5,13.5,13.5,13.5,13.5,13.5,13.5,13.5,13.5,13.5;", "set 5GHz.Target.Power.Vht80[1]=13.5,13.5,13.5,13.5,13.5,13.5,13.5,13.5,13.5,13.5,13.5,13.5,13.5,13.5,13.5,13.5,13.5,13.5,13.5,13.5,13.5,13.5,13.5,13.5;", "set 5GHz.Target.Power.Vht80[2]=13.5,13.5,13.5,13.5,13.5,13.5,13.5,13.5,13.5,13.5,13.5,13.5,13.5,13.5,13.5,13.5,13.5,13.5,13.5,13.5,13.5,13.5,13.5,13.5;", "set 5GHz.Target.Power.Vht80[3]=19,19,18,17,17,16,14,14,19,19,18,17,17,16,14,14,19,19,18,17,17,16,14,14;", "set 5GHz.Target.Power.Vht80[4]=19,19,18,17,17,16,14,14,19,19,18,17,17,16,14,14,19,19,18,17,17,16,14,14;", "set 5GHz.Target.Power.Vht80[5]=19,19,18,17,17,16,14,14,19,19,18,17,17,16,14,14,19,19,18,17,17,16,14,14;", "setcal dll=cal-2p;", "setcal scheme=2;", "setcal PowerGoalMode=1;", "setcal 5gfreq=5180,5240,5320,5520,5640,5745,5785,5825;", "setcal 5gGainIndex1Ch0=9,9,9,9,9,9,10,10;", "setcal 5gGainIndex1Ch1=9,9,9,9,9,9,10,10;", "setcal 5gGainIndex1Ch2=9,9,9,9,9,9,10,10;", "setcal 5gDacGain1=0,0,0,0,0,0,0,0;", "setcal 5gPowerGoal1=14.0,14.0,14.0,14.0,14.0,14.0,14.0,14.0;", "setcal 5gGainIndex2Ch0=12,12,12,12,12,12,13,13;", "setcal 5gGainIndex2Ch1=12,12,12,12,12,12,13,13;", "setcal 5gGainIndex2Ch2=12,12,12,12,12,12,13,13;", "setcal 5gDacGain2=-6,-6,-6,-6,-6,-6,-6,-6;", "setcal 5gPowerGoal2=14.0,14.0,14.0,14.0,14.0,14.0,14.0,14.0;", "set customer=cus223-022-n0624;", "set 5GHz.Target.Frequency.Legacy[0]=5180;", "set 5GHz.Target.Frequency.Legacy[1]=5240;", "set 5GHz.Target.Frequency.Legacy[2]=5320;", "set 5GHz.Target.Frequency.Legacy[3]=5500;", "set 5GHz.Target.Frequency.Legacy[4]=5600;", "set 5GHz.Target.Frequency.Legacy[5]=5745;"] ("最终指令")) -> ()  [unwired: 1 out]
  n2 = Index Array(array=w1, index="index") -> (element=→"Cmd":string)
  n3 = Array Size(array=w1) -> (size(s)=→"CmdCount":i32)
  n4 = disable-structure shown="Disabled" {
    frame Disabled {
      (unwired) string[] [" load memory=otp;", " hello", " set customer=WB335B;", " template prefer=4; allow=4,2; install=yes;", " set ssid=3027;", " set svid=168c;", " set config=1;address=407c;", " set config=18212ede;address=18c00;", " set config=000801d8;address=18c04;", " set config=0003780c;address=18c08;", " set devicetype=5;", " set regdmn=6A;", " Set txmask=1;", " Set rxmask=1;", " set opflags=2;", " set antctrlcommon2g=400550;", " set antctrlcommon22g=22222;", " set antCtrlChain2g=150,150,10;", " set antctrlcommon5g=400550;", " set antctrlcommon25g=22222;", " set antCtrlChain5g=150,150,10;", " set xatten1Margin2g=0,0,0;", " set xatten1Margin5g=0,0,0;", " set xatten1Marginlow5g=0,0,0;", " set xatten1Marginhigh5g=0,0,0;", " set xatten1db2g=0,0,0;", " set xatten1db5g=0,0,0;", " set xatten1dblow5g=0,0,0;", " set xatten1dbhigh5g=0,0,0;", " set switchcomspdt2g=353;", " set switchcomspdt5g=393;", " set txgainTable=1;", " set rxgainTable=1;", " set temperatureCompensation=1;", " set tempSlope2g=25;", " set tempSlope5g=55;", " set tempSlopelow=45;", " set tempSlopehigh=60;", " set thermometer=0;", " set eepromWriteEnable=10;", " set spurchans2g=2440,2464,2480,0,0;", " set spurchans5g=5200,5520,5600,5680,5800;", " set swregenable=1;", " set swreg=0x121e4276;", " set papdenable=0;", " set papd2gRateMaskHt20=0x0800ffff;", " set papd2gRateMaskHt40=0x0800ffff;", " set 2GHz.Target.Frequency.Cck=2412,2472;", " set 2GHz.Target.Power.Cck[0]=18,18,18,18;", " set 2GHz.Target.Power.Cck[1]=18,18,18,18;", " set 2GHz.Target.Frequency.Legacy=2412,2437,2472;", " set 2GHz.Target.Power.Legacy[0]=18,17,16,14;", " set 2GHz.Target.Power.Legacy[1]=18,17,16,14;", " set 2GHz.Target.Power.Legacy[2]=18,17,16,14;", " set 2GHz.Target.Frequency.Ht20=2412,2437,2472;", " set 2GHz.Target.Power.Ht20[0]=17,17,17,16,15,13,0,0,0,0,0,0,0,0;", " set 2GHz.Target.Power.Ht20[1]=17,17,17,16,15,13,0,0,0,0,0,0,0,0;", " set 2GHz.Target.Power.Ht20[2]=17,17,17,16,15,13,0,0,0,0,0,0,0,0;", " set 2GHz.Target.Frequency.Ht40=2412,2437,2452;", " set 2GHz.Target.Power.Ht40[0]=16,16,16,16,15,13,0,0,0,0,0,0,0,0;", " set 2GHz.Target.Power.Ht40[1]=16,16,16,16,15,13,0,0,0,0,0,0,0,0;", " set 2GHz.Target.Power.Ht40[2]=16,16,16,16,15,13,0,0,0,0,0,0,0,0;", " set caltgtfreq5g=5180,5240,5320,5400,5500,5600,5700,5825;", " set caltgtpwr5g[0]=15,14,13,10;", " set caltgtpwr5g[1]=15,14,13,10;", " set caltgtpwr5g[2]=15,14,13,10;", " set caltgtpwr5g[3]=15,14,13,10;", " set caltgtpwr5g[4]=14,13,12,9;", " set caltgtpwr5g[5]=14,13,12,9;", " set caltgtpwr5g[6]=14,13,12,8;", " set caltgtpwr5g[7]=14,13,12,8;", " set caltgtfreqht205g=5180,5240,5320,5400,5500,5700,5745,5825;", " set caltgtpwrht205g[0]=14,13,12,11,10,9,0,0,0,0,0,0,0,0;", " set caltgtpwrht205g[1]=14,13,12,11,10,9,0,0,0,0,0,0,0,0;", " set caltgtpwrht205g[2]=14,13,12,11,10,9,0,0,0,0,0,0,0,0;", " set caltgtpwrht205g[3]=14,13,12,11,10,9,0,0,0,0,0,0,0,0;", " set caltgtpwrht205g[4]=14,13,12,11,10,9,0,0,0,0,0,0,0,0;", " set caltgtpwrht205g[5]=14,13,12,11,10,9,0,0,0,0,0,0,0,0;", " set caltgtpwrht205g[6]=14,13,12,11,10,9,0,0,0,0,0,0,0,0;", " set caltgtpwrht205g[7]=14,13,12,11,10,9,0,0,0,0,0,0,0,0;", " set caltgtfreqht405g=5180,5240,5320,5400,5500,5700,5745,5785;", " set caltgtpwrht405g[0]=14,13,12,11,10,9,0,0,0,0,0,0,0,0;", " set caltgtpwrht405g[1]=14,13,12,11,10,9,0,0,0,0,0,0,0,0;", " set caltgtpwrht405g[2]=14,13,12,11,10,9,0,0,0,0,0,0,0,0;", " set caltgtpwrht405g[3]=14,13,12,11,10,9,0,0,0,0,0,0,0,0;", " set caltgtpwrht405g[4]=14,13,12,11,10,9,0,0,0,0,0,0,0,0;", " set caltgtpwrht405g[5]=14,13,12,11,10,9,0,0,0,0,0,0,0,0;", " set caltgtpwrht405g[6]=14,13,12,11,10,9,0,0,0,0,0,0,0,0;", " set caltgtpwrht405g[7]=14,13,12,11,10,9,0,0,0,0,0,0,0,0;", " set rfsilent=0;", " set rfsilent=2D;", " set config=3a000400;address=4014;", " set config=ffc25001;address=5040;", " set tempslopextension=1;", " set tempSlopeExtension=45,45,50,50,60,55,60,60;", " set 2GHz.ctl.Index[0]=0x11;", " set 2GHz.ctl.Frequency[0]=2412,2417,2457,2462;", " set 2GHz.ctl.Power[0]=17.5,18  ,18  ,17.5;", " set 2GHz.ctl.BandEdge[0]=0   ,1   ,0   ,0;", " set 2GHz.ctl.Index[1]=0x12;", " set 2GHz.ctl.Frequency[1]=2412,2417,2422,2457;", " set 2GHz.ctl.Power[1]=12  ,17  ,18  ,15;", " set 2GHz.ctl.BandEdge[1]=0   ,0   ,1   ,1;", " set 2GHz.ctl.Index[2]=0x15;", " set 2GHz.ctl.Frequency[2]=2412,2417,2457,2462;", " set 2GHz.ctl.Power[2]=11  ,16.5,16.5,13.5;", " set 2GHz.ctl.BandEdge[2]=0   ,1   ,0   ,0;", " set 2GHz.ctl.Index[3]=0x17;", " set 2GHz.ctl.Frequency[3]=2422,2427,2432,2452;", " set 2GHz.ctl.Power[3]=11  ,13  ,14.5,12;", " set 2GHz.ctl.BandEdge[3]=0   ,0   ,1   ,0;", " set 2GHz.ctl.Index[4]=0x41;", " set 2GHz.ctl.Frequency[4]=2412,2417,2472,2484;", " set 2GHz.ctl.Power[4]=18  ,18  ,18  ,18;", " set 2GHz.ctl.BandEdge[4]=0   ,1   ,0   ,0;", " set 2GHz.ctl.Index[5]=0x42;", " set 2GHz.ctl.Frequency[5]=2412,2417,2467,2472;", " set 2GHz.ctl.Power[5]=18  ,18  ,18  ,18;", " set 2GHz.ctl.BandEdge[5]=0   ,1   ,0   ,0;", " set 2GHz.ctl.Index[6]=0x45;", " set 2GHz.ctl.Frequency[6]=2412,2417,2467,2472;", " set 2GHz.ctl.Power[6]=16  ,16  ,16  ,16;", " set 2GHz.ctl.BandEdge[6]=0   ,1   ,0   ,0;", " set 2GHz.ctl.Index[7]=0x47;", " set 2GHz.ctl.Frequency[7]=2422,2427,2457,2462;", " set 2GHz.ctl.Power[7]=15  ,15  ,15  ,15;", " set 2GHz.ctl.BandEdge[7]=0   ,1   ,0   ,0;", " set 2GHz.ctl.Index[8]=0x31;", " set 2GHz.ctl.Frequency[8]=2412,2417,2467,2472;", " set 2GHz.ctl.Power[8]=15.5,16  ,16  ,15.5;", " set 2GHz.ctl.BandEdge[8]=0   ,1   ,0   ,0;", " set 2GHz.ctl.Index[9]=0x32;", " set 2GHz.ctl.Frequency[9]=2412,2417,2467,2472;", " set 2GHz.ctl.Power[9]=15.5,16  ,16  ,15.5;", " set 2GHz.ctl.BandEdge[9]=0   ,1   ,0   ,0;", " set 2GHz.ctl.Index[10]=0x35;", " set 2GHz.ctl.Frequency[10]=2412,2417,2467,2472;", " set 2GHz.ctl.Power[10]=15.5,16  ,16  ,15.5;", " set 2GHz.ctl.BandEdge[10]=0   ,1   ,0   ,0;", " set 2GHz.ctl.Index[11]=0x37;", " set 2GHz.ctl.Frequency[11]=2422,2427,2457,2462;", " set 2GHz.ctl.Power[11]=15.5,15.5,15.5,15.5;", " set 2GHz.ctl.BandEdge[11]=0   ,1   ,0   ,0;", " set config=00036c11;address=507c;", " set config=05048dc0;address=5074;", " set config=102021b;address=4004;", " set config=1;address=407c;", " set config=36168c;address=5000;", " set config=2800001;address=5008;", " set config=173f3f01;address=570c;", " or2 bank=0; size=1; a=+47;", " or2 bank=0; size=1; a=+73;", " or2 bank=1; size=1; a=+3;", " ow2 bank=0; size=1; a=13a; v=14;", " ow2 bank=0; size=1; a=13b; v=40;", " ow2 bank=0;size=1;a=+307;v=5c;", " fw a=63120[8,7]; v=0;", " ow bank=0; size=2; a=+114; v=8020;", " ow bank=0; size=1; a=+116; v=00;", " ow bank=0; size=1; a=+117; v=74;", " ow bank=0; size=2; a=+118; v=5597;", " ow bank=0; size=1; a=+120; v=00;", " ow bank=0; size=2; a=+121; v=8220;", " ow bank=0; size=1; a=+123; v=00;", " ow bank=0; size=4; a=+124; v=00000001;", " ow bank=0; size=1; a=+293; v=20;", " ow bank=0; size=2; a=+294; v=0084;", " ow bank=0; size=4; a=+296; v=A505ad10;", " ow bank=0; size=2; a=+112; v=dace;", " set mac=24:fd:52:22:3b:3c;", " set customer=WB335B;", "reset"]  # ART2 138 Initial CMD For WB335B - 20130722
      (unwired) string[] [" load memory=otp;", " hello", " set customer=WB335B;", " template prefer=4; allow=4,2; install=yes;", " set ssid=3027;", " set svid=168c;", " set config=1;address=407c;", " set config=18212ede;address=18c00;", " set config=000801d8;address=18c04;", " set config=0003780c;address=18c08;", " set devicetype=5;", " set regdmn=0;", " Set txmask=1;", " Set rxmask=1;", " set opflags=2;", " set antctrlcommon2g=400550;", " set antctrlcommon22g=22222;", " set antCtrlChain2g=150,150,10;", " set antctrlcommon5g=400550;", " set antctrlcommon25g=22222;", " set antCtrlChain5g=150,150,10;", " set xatten1Margin2g=0,0,0;", " set xatten1Margin5g=0,0,0;", " set xatten1Marginlow5g=0,0,0;", " set xatten1Marginhigh5g=0,0,0;", " set xatten1db2g=0,0,0;", " set xatten1db5g=0,0,0;", " set xatten1dblow5g=0,0,0;", " set xatten1dbhigh5g=0,0,0;", " set switchcomspdt2g=353;", " set switchcomspdt5g=393;", " set antDivCtrl=0xC9;", " set txgainTable=1;", " set rxgainTable=1;", " set temperatureCompensation=1;", " set tempSlope2g=25;", " set tempSlope5g=55;", " set tempSlopelow=45;", " set tempSlopehigh=60;", " set thermometer=0;", " set eepromWriteEnable=10;", " set spurchans2g=2440,2464,2480,0,0;", " set spurchans5g=5200,5520,5600,5680,5800;", " set swregenable=1;", " set swreg=0x121e4276;", " set papdenable=0;", " set papd2gRateMaskHt20=0x0800ffff;", " set papd2gRateMaskHt40=0x0800ffff;", " set 2GHz.Target.Frequency.Cck=2412,2472;", " set 2GHz.Target.Power.Cck[0]=18,18,18,18;", " set 2GHz.Target.Power.Cck[1]=18,18,18,18;", " set 2GHz.Target.Frequency.Legacy=2412,2437,2472;", " set 2GHz.Target.Power.Legacy[0]=18,17,16,14;", " set 2GHz.Target.Power.Legacy[1]=18,17,16,14;", " set 2GHz.Target.Power.Legacy[2]=18,17,16,14;", " set 2GHz.Target.Frequency.Ht20=2412,2437,2472;", " set 2GHz.Target.Power.Ht20[0]=17,17,17,16,15,13,0,0,0,0,0,0,0,0;", " set 2GHz.Target.Power.Ht20[1]=17,17,17,16,15,13,0,0,0,0,0,0,0,0;", " set 2GHz.Target.Power.Ht20[2]=17,17,17,16,15,13,0,0,0,0,0,0,0,0;", " set 2GHz.Target.Frequency.Ht40=2412,2437,2452;", " set 2GHz.Target.Power.Ht40[0]=16,16,16,16,15,13,0,0,0,0,0,0,0,0;", " set 2GHz.Target.Power.Ht40[1]=16,16,16,16,15,13,0,0,0,0,0,0,0,0;", " set 2GHz.Target.Power.Ht40[2]=16,16,16,16,15,13,0,0,0,0,0,0,0,0;", " set caltgtfreq5g=5180,5240,5320,5400,5500,5600,5700,5825;", " set caltgtpwr5g[0]=15,14,13,10;", " set caltgtpwr5g[1]=15,14,13,10;", " set caltgtpwr5g[2]=15,14,13,10;", " set caltgtpwr5g[3]=15,14,13,10;", " set caltgtpwr5g[4]=14,13,12,9;", " set caltgtpwr5g[5]=14,13,12,9;", " set caltgtpwr5g[6]=14,13,12,8;", " set caltgtpwr5g[7]=14,13,12,8;", " set caltgtfreqht205g=5180,5240,5320,5400,5500,5700,5745,5825;", " set caltgtpwrht205g[0]=14,13,12,11,10,9,0,0,0,0,0,0,0,0;", " set caltgtpwrht205g[1]=14,13,12,11,10,9,0,0,0,0,0,0,0,0;", " set caltgtpwrht205g[2]=14,13,12,11,10,9,0,0,0,0,0,0,0,0;", " set caltgtpwrht205g[3]=14,13,12,11,10,9,0,0,0,0,0,0,0,0;", " set caltgtpwrht205g[4]=14,13,12,11,10,9,0,0,0,0,0,0,0,0;", " set caltgtpwrht205g[5]=14,13,12,11,10,9,0,0,0,0,0,0,0,0;", " set caltgtpwrht205g[6]=14,13,12,11,10,9,0,0,0,0,0,0,0,0;", " set caltgtpwrht205g[7]=14,13,12,11,10,9,0,0,0,0,0,0,0,0;", " set caltgtfreqht405g=5180,5240,5320,5400,5500,5700,5745,5785;", " set caltgtpwrht405g[0]=14,13,12,11,10,9,0,0,0,0,0,0,0,0;", " set caltgtpwrht405g[1]=14,13,12,11,10,9,0,0,0,0,0,0,0,0;", " set caltgtpwrht405g[2]=14,13,12,11,10,9,0,0,0,0,0,0,0,0;", " set caltgtpwrht405g[3]=14,13,12,11,10,9,0,0,0,0,0,0,0,0;", " set caltgtpwrht405g[4]=14,13,12,11,10,9,0,0,0,0,0,0,0,0;", " set caltgtpwrht405g[5]=14,13,12,11,10,9,0,0,0,0,0,0,0,0;", " set caltgtpwrht405g[6]=14,13,12,11,10,9,0,0,0,0,0,0,0,0;", " set caltgtpwrht405g[7]=14,13,12,11,10,9,0,0,0,0,0,0,0,0;", " set rfsilent=0;", " set rfsilent=2D;", " set config=3a000400;address=4014;", " set config=ffc25001;address=5040;", " set tempslopextension=1;", " set tempSlopeExtension=45,45,50,50,60,55,60,60;", " set 2GHz.ctl.Index[0]=0x11;", " set 2GHz.ctl.Frequency[0]=2412,2417,2457,2462;", " set 2GHz.ctl.Power[0]=17.5,18  ,18  ,17.5;", " set 2GHz.ctl.BandEdge[0]=0   ,1   ,0   ,0;", " set 2GHz.ctl.Index[1]=0x12;", " set 2GHz.ctl.Frequency[1]=2412,2417,2422,2457;", " set 2GHz.ctl.Power[1]=12  ,17  ,18  ,15;", " set 2GHz.ctl.BandEdge[1]=0   ,0   ,1   ,1;", " set 2GHz.ctl.Index[2]=0x15;", " set 2GHz.ctl.Frequency[2]=2412,2417,2457,2462;", " set 2GHz.ctl.Power[2]=11  ,16.5,16.5,13.5;", " set 2GHz.ctl.BandEdge[2]=0   ,1   ,0   ,0;", " set 2GHz.ctl.Index[3]=0x17;", " set 2GHz.ctl.Frequency[3]=2422,2427,2432,2452;", " set 2GHz.ctl.Power[3]=11  ,13  ,14.5,12;", " set 2GHz.ctl.BandEdge[3]=0   ,0   ,1   ,0;", " set 2GHz.ctl.Index[4]=0x41;", " set 2GHz.ctl.Frequency[4]=2412,2417,2472,2484;", " set 2GHz.ctl.Power[4]=18  ,18  ,18  ,18;", " set 2GHz.ctl.BandEdge[4]=0   ,1   ,0   ,0;", " set 2GHz.ctl.Index[5]=0x42;", " set 2GHz.ctl.Frequency[5]=2412,2417,2467,2472;", " set 2GHz.ctl.Power[5]=18  ,18  ,18  ,18;", " set 2GHz.ctl.BandEdge[5]=0   ,1   ,0   ,0;", " set 2GHz.ctl.Index[6]=0x45;", " set 2GHz.ctl.Frequency[6]=2412,2417,2467,2472;", " set 2GHz.ctl.Power[6]=16  ,16  ,16  ,16;", " set 2GHz.ctl.BandEdge[6]=0   ,1   ,0   ,0;", " set 2GHz.ctl.Index[7]=0x47;", " set 2GHz.ctl.Frequency[7]=2422,2427,2457,2462;", " set 2GHz.ctl.Power[7]=15  ,15  ,15  ,15;", " set 2GHz.ctl.BandEdge[7]=0   ,1   ,0   ,0;", " set 2GHz.ctl.Index[8]=0x31;", " set 2GHz.ctl.Frequency[8]=2412,2417,2467,2472;", " set 2GHz.ctl.Power[8]=15.5,16  ,16  ,15.5;", " set 2GHz.ctl.BandEdge[8]=0   ,1   ,0   ,0;", " set 2GHz.ctl.Index[9]=0x32;", " set 2GHz.ctl.Frequency[9]=2412,2417,2467,2472;", " set 2GHz.ctl.Power[9]=15.5,16  ,16  ,15.5;", " set 2GHz.ctl.BandEdge[9]=0   ,1   ,0   ,0;", " set 2GHz.ctl.Index[10]=0x35;", " set 2GHz.ctl.Frequency[10]=2412,2417,2467,2472;", " set 2GHz.ctl.Power[10]=15.5,16  ,16  ,15.5;", " set 2GHz.ctl.BandEdge[10]=0   ,1   ,0   ,0;", " set 2GHz.ctl.Index[11]=0x37;", " set 2GHz.ctl.Frequency[11]=2422,2427,2457,2462;", " set 2GHz.ctl.Power[11]=15.5,15.5,15.5,15.5;", " set 2GHz.ctl.BandEdge[11]=0   ,1   ,0   ,0;", " set config=00036c11;address=507c;", " set config=05048dc0;address=5074;", " set config=102021b;address=4004;", " set config=1;address=407c;", " set config=36168c;address=5000;", " set config=2800001;address=5008;", " set config=173f3f01;address=570c;", " or2 bank=0; size=1; a=+47;", " or2 bank=0; size=1; a=+73;", " or2 bank=1; size=1; a=+3;", " ow2 bank=0; size=1; a=13a; v=14;", " ow2 bank=0; size=1; a=13b; v=40;", " fw a=63120[8,7]; v=0;", " ow bank=0; size=2; a=+114; v=8020;", " ow bank=0; size=1; a=+116; v=00;", " ow bank=0; size=1; a=+117; v=74;", " ow bank=0; size=2; a=+118; v=5597;", " ow bank=0; size=1; a=+120; v=00;", " ow bank=0; size=2; a=+121; v=8220;", " ow bank=0; size=1; a=+123; v=00;", " ow bank=0; size=4; a=+124; v=00000001;", " ow bank=0; size=1; a=+293; v=20;", " ow bank=0; size=2; a=+294; v=0084;", " ow bank=0; size=4; a=+296; v=A505ad10;", " ow bank=0; size=2; a=+112; v=dace;", " set mac=24:fd:52:22:3b:3c;", " set customer=WB335B;", "reset"]  # ART2 138 Initial CMD For WB335B - Howard
      (unwired) string[] ["hello", "load", "template prefer=4; allow=4,2; install=yes;", "set ssid=411c;", "set svid=144d;", "set config=1;address=407c", "set config=18212ede;address=18c00", "set config=000801d8;address=18c04", "set config=0003780c;address=18c08", "set customer=WB335-010-D0001", "set devicetype=5", "set regdmn=6a", "Set txmask=1;", "Set rxmask=1;", "set opflags=2;", "set antctrlcommon2g=400550;", "set antctrlcommon22g=22222;", "set antCtrlChain2g=150,150,10;", "set antctrlcommon5g=400550;", "set antctrlcommon25g=22222;", "set antCtrlChain5g=150,150,10;", "set xatten1Margin2g=0,0,0;", "set xatten1Margin5g=0,0,0;", "set xatten1Marginlow5g=0,0,0;", "set xatten1Marginhigh5g=0,0,0;", "set xatten1db2g=0,0,0;", "set xatten1db5g=0,0,0;", "set xatten1dblow5g=0,0,0;", "set xatten1dbhigh5g=0,0,0;", "set switchcomspdt2g=353;", "set switchcomspdt5g=393;", "set txgainTable=1;", "set rxgainTable=1;", "set temperatureCompensation=1", "set tempSlope2g=25", "set tempSlope5g=55", "set tempSlopelow=45", "set tempSlopehigh=60", "set thermometer=0;", "set eepromWriteEnable=10;", "set spurchans2g=2440,2464,2480,0,0;", "set spurchans5g=5200,5520,5600,5680,5800;", "set swregenable=1;", "set swreg=0x121e4276;", "set papdenable=0;", "set papd2gRateMaskHt20=0x0800ffff;", "set papd2gRateMaskHt40=0x0800ffff;", "set  2GHz.Target.Frequency.Cck=2412,2472;", "set  2GHz.Target.Power.Cck[0]=17,17,17,17;", "set  2GHz.Target.Power.Cck[1]=17,17,17,17;", "set  2GHz.Target.Frequency.Legacy=2412,2437, 2472;", "set  2GHz.Target.Power.Legacy[0]=18,17,16,14;", "set  2GHz.Target.Power.Legacy[1]=18,17,16,14;", "set  2GHz.Target.Power.Legacy[2]=18,17,16,14;", "set  2GHz.Target.Frequency.Ht20=2412,2437, 2472;", "set  2GHz.Target.Power.Ht20[0]=16,16,16,16,15,13,0,0,0,0,0,0,0,0;", "set  2GHz.Target.Power.Ht20[1]=16,16,16,16,15,13,0,0,0,0,0,0,0,0;", "set  2GHz.Target.Power.Ht20[2]=16,16,16,16,15,13,0,0,0,0,0,0,0,0;", "set  2GHz.Target.Frequency.Ht40=2412,2437, 2452;", "set  2GHz.Target.Power.Ht40[0]=16,16,16,16,15,13,0,0,0,0,0,0,0,0;", "set  2GHz.Target.Power.Ht40[1]=16,16,16,16,15,13,0,0,0,0,0,0,0,0;", "set  2GHz.Target.Power.Ht40[2]=16,16,16,16,15,13,0,0,0,0,0,0,0,0;", "set caltgtfreq5g=5180,5240,5320,5400,5500,5600,5700,5825;", "set caltgtpwr5g=v.(15,14,13,10),f.0;", "set caltgtpwr5g=v.(15,14,13,10),f.1;", "set caltgtpwr5g=v.(15,14,13,10),f.2;", "set caltgtpwr5g=v.(15,14,13,10),f.3;", "set caltgtpwr5g=v.(14,13,12,9),f.4;", "set caltgtpwr5g=v.(14,13,12,9),f.5;", "set caltgtpwr5g=v.(14,13,12,8),f.6;", "set caltgtpwr5g=v.(14,13,12,8),f.7;", "set caltgtfreqht205g=5180,5240,5320,5400,5500,5700,5745,5825;", "set caltgtpwrht205g=v.(14,13,12,11,10,9,0,0,0,0,0,0,0,0),f.0;", "set caltgtpwrht205g=v.(14,13,12,11,10,9,0,0,0,0,0,0,0,0),f.1;", "set caltgtpwrht205g=v.(14,13,12,11,10,9,0,0,0,0,0,0,0,0),f.2;", "set caltgtpwrht205g=v.(14,13,12,11,10,9,0,0,0,0,0,0,0,0),f.3;", "set caltgtpwrht205g=v.(14,13,12,11,10,9,0,0,0,0,0,0,0,0),f.4;", "set caltgtpwrht205g=v.(14,13,12,11,10,9,0,0,0,0,0,0,0,0),f.5;", "set caltgtpwrht205g=v.(14,13,12,11,10,9,0,0,0,0,0,0,0,0),f.6;", "set caltgtpwrht205g=v.(14,13,12,11,10,9,0,0,0,0,0,0,0,0),f.7;", "set caltgtfreqht405g=5180,5240,5320,5400,5500,5700,5745,5785;", "set caltgtpwrht405g=v.(14,13,12,11,10,9,0,0,0,0,0,0,0,0),f.0;", "set caltgtpwrht405g=v.(14,13,12,11,10,9,0,0,0,0,0,0,0,0),f.1;", "set caltgtpwrht405g=v.(14,13,12,11,10,9,0,0,0,0,0,0,0,0),f.2;", "set caltgtpwrht405g=v.(14,13,12,11,10,9,0,0,0,0,0,0,0,0),f.3;", "set caltgtpwrht405g=v.(14,13,12,11,10,9,0,0,0,0,0,0,0,0),f.4;", "set caltgtpwrht405g=v.(14,13,12,11,10,9,0,0,0,0,0,0,0,0),f.5;", "set caltgtpwrht405g=v.(14,13,12,11,10,9,0,0,0,0,0,0,0,0),f.6;", "set caltgtpwrht405g=v.(14,13,12,11,10,9,0,0,0,0,0,0,0,0),f.7;", "set rfsilent=0;", "set rfsilent=2D;", "set  config=3a000400; address=4014;", "set  config=ffc25001; address=5040;", "set tempslopextension=1", "set tempSlopeExtension=45,45,50,50,60,55,60,60;", "set  2GHz.ctl.Index[0]=0x11;", "set  2GHz.ctl.Frequency[0]=2412,2417,2457,2462;", "set  2GHz.ctl.Power[0]=    18  ,18  ,18  ,17;", "set  2GHz.ctl.BandEdge[0]= 0   ,1   ,0   , 0;", "set  2GHz.ctl.Index[1]=0x12;", "set  2GHz.ctl.Frequency[1]=2412,2417,2457,2462;", "set  2GHz.ctl.Power[1]=    13.5,16.5,15.5,13.5;", "set  2GHz.ctl.BandEdge[1]= 0   ,0   ,0   ,0;", "set  2GHz.ctl.Index[2]=0x15;", "set  2GHz.ctl.Frequency[2]=2412,2417,2457,2462;", "set  2GHz.ctl.Power[2]=    13  ,16  ,15.5,13;", "set  2GHz.ctl.BandEdge[2]= 0   ,0   ,0   ,0;", "set  2GHz.ctl.Index[3]=0x17;", "set  2GHz.ctl.Frequency[3]=2422,2427,2447,2452;", "set  2GHz.ctl.Power[3]=    10  ,11.5,12.5,11.5;", "set  2GHz.ctl.BandEdge[3]= 0   ,0   ,0  ,0;", "set  2GHz.ctl.Index[4]=0x41;", "set  2GHz.ctl.Frequency[4]=2412,2472,2484,2484;", "set  2GHz.ctl.Power[4]=    17.5,17.5,18,18;", "set  2GHz.ctl.BandEdge[4]= 1   ,0   ,0   ,0;", "set  2GHz.ctl.Index[5]=0x42;", "set  2GHz.ctl.Frequency[5]=2412,2417,2472,2472;", "set  2GHz.ctl.Power[5]=    17.5,18  ,17.5,17.5;", "set  2GHz.ctl.BandEdge[5]= 0   ,1   ,0   ,0;", "set  2GHz.ctl.Index[6]=0x45;", "set  2GHz.ctl.Frequency[6]=2412,2472,2472,2472;", "set  2GHz.ctl.Power[6]=    17.5,17.5,17.5,17.5;", "set  2GHz.ctl.BandEdge[6]= 1   ,0   ,0   ,0;", "set  2GHz.ctl.Index[7]=0x47;", "set  2GHz.ctl.Frequency[7]=2422,2427,2457,2462;", "set  2GHz.ctl.Power[7]=    16  ,16.5,16.5,16;", "set  2GHz.ctl.BandEdge[7]= 0   ,1   ,0   ,0;", "set  2GHz.ctl.Index[8]=0x31;", "set  2GHz.ctl.Frequency[8]=2412,2472,2472,2472;", "set  2GHz.ctl.Power[8]=    15  ,15  ,15  ,15;", "set  2GHz.ctl.BandEdge[8]= 1   ,0   ,0   ,0;", "set  2GHz.ctl.Index[9]=0x32;", "set  2GHz.ctl.Frequency[9]=2412,2417,2472,2472;", "set  2GHz.ctl.Power[9]=    14  ,15.5,13 ,13;", "set  2GHz.ctl.BandEdge[9]= 0   ,1   ,0   ,0;", "set  2GHz.ctl.Index[10]=0x35;", "set  2GHz.ctl.Frequency[10]=2412,2417,2467,2472;", "set  2GHz.ctl.Power[10]=    14  ,15.5,15.5,13;", "set  2GHz.ctl.BandEdge[10]= 0   ,1   ,0   ,0;", "set  2GHz.ctl.Index[11]=0x37;", "set  2GHz.ctl.Frequency[11]=2422,2427,2457,2462;", "set  2GHz.ctl.Power[11]=    14.5,16  ,16  ,14.5;", "set  2GHz.ctl.BandEdge[11]= 0   ,1   ,0   ,0;", "set  config=00036c11; address=507c;", "set  config=05048dc0; address=5074;", "set config=102021b; address=4004;", "set config=1; address=407c;", "set config=36168c; address=5000;", "set config=2800001; address=5008;", "set config=173f3f01; address=570c;", "rr a=6310c;", "get regdmn", "or2 bank=0;size=1;a=+47;", "or2 bank=0;size=1;a=+73;", "ow2 bank=0;size=1;a=+44;v=13", "ow2 bank=0;size=1;a=+45;v=64", "ow2 bank=0;size=1;a=+46;v=66", "ow2 bank=0;size=1;a=+47;v=22", "ow2 bank=0;size=1;a=+60;v=1F", "ow2 bank=0;size=1;a=+61;v=08", "ow2 bank=0;size=1;a=+62;v=04", "ow2 bank=0;size=1;a=+63;v=00", "ow2 bank=0;size=1;a=+73;v=2C", "rw a=44000;v=40100;", "rr a=44000;", "or2 bank=1;size=1;a=+3;", "rw a=20104;v=81313332;", "rw a=20104;v=C1313332;", "rw a=20104;v=C1313333;", "rw a=63280;v=4081F;", "rw a=63284;v=104CCCCC;", "rw a=20104;v=C1313332;", "rw a=20104;v=81313332;", "fw a=63120[8,7];v=0;", "rr a=4020;", "get regdmn", "or2 bank=0;size=2;a=0x70;", "ow bank=0;size=2;a=+114;v=8020;", "ow bank=0;size=1;a=+116;v=00;", "or2 bank=0;size=2;a=+114;", "or2 bank=0;size=1;a=+116;", "ow bank=0;size=1;a=+117;v=74;", "ow bank=0;size=2;a=+118;v=5597;", "ow bank=0;size=1;a=+120;v=00;", "or2 bank=0;size=1;a=+117;", "or2 bank=0;size=2;a=+118;", "or2 bank=0;size=1;a=+120;", "ow bank=0;size=2;a=+121;v=8220;", "ow bank=0;size=1;a=+123;v=00;", "ow bank=0;size=4;a=+124;v=00000001;", "or2 bank=0;size=2;a=+121;", "or2 bank=0;size=1;a=+123;", "or2 bank=0;size=4;a=+124;", "ow bank=0;size=1;a=+293;v=20;", "ow bank=0;size=2;a=+294;v=0084;", "ow bank=0;size=4;a=+296;v=A505ad10;", "or2 bank=0;size=1;a=+293;", "or2 bank=0;size=2;a=+294;", "or2 bank=0;size=4;a=+296;", "ow bank=0;size=2;a=+112;v=dace;", "or2 bank=0;size=2;a=+112;", "rr a=4020;", "get regdmn", "or2 bank=0;a=13a;size=2;", "ow2 bank=0;size=1;a=13a;v=14", "or2 bank=0;size=1;a=13a;", "ow2 bank=0;size=1;a=13b;v=40", "or2 bank=0;size=1;a=13b;", "or2 bank=0;a=13c;size=2;", "ow2 bank=0;size=1;a=13c;v=14", "or2 bank=0;size=1;a=13c;", "ow2 bank=0;size=1;a=13d;v=40", "or2 bank=0;size=1;a=13d;", "or bank=0;size=1;a=c", "or bank=0;size=1;a=e", "ow bank=0;size=1;a=c;v=2", "or bank=0;size=1;a=c", "ow bank=0;size=1;a=e;v=37", "ow bank=0;size=1;a=f;v=1a", "or bank=0;size=1;a=e", "set config=00000000; address=500c;", "set config=00000003; address=35044;", "set config=5bc35001; address=35040;", "rr a=4020;", "get regdmn", "set config=00010000; address=35050;", "set config=00000066; address=44014;", "set config=01FF0000; address=20100;", "set config=0000000c; address=20120;", "set config=00000008; address=20120;", "set config=00000062; address=44014;", "set config=10110003; address=35080;", "or2 bank=1;size=1;a=+3;", "ow bank=1;size=4;a=0;v=04000000;", "sw a=BB_scrambler_seed.fixed_scrambler_seed;v=1", "sw a=BB_phyonly_control.generate_scrambler;v=0", "reset"]  # Litepoint ART 147 Initial CMD for WB335B
    }
    frame Enabled {
    }
  }
  "error out" <- "error in (no error)"
  "Command List" <- w1
